vi "setMagnet.vi"(4 "Mode":T2, 6 "Axis":T1=enum."Z", 8 "error in (no error)":errorcluster, 9 "Target Rate (T/min)":dbl, 10 "Target Field (T)":dbl, 11 "Instrument.Cryostat in":refnum<class "Instrument.Cryostat.lvclass">) -> (0 "error out":errorcluster, 3 "Instrument.Cryostat out":refnum<class "Instrument.Cryostat.lvclass">)   [LabVIEW 2019, in "Instrument.Cryostat.lvclass"]
uses:
  Instrument.Cryostat.lvclass
  Typedefs/Magnet Mode--Enum.ctl
  Typedefs/Magnet Axis--Enum.ctl
  Typedefs/setMagnet--cluster.ctl
  Typedefs/Cryostat.commands--enum.ctl
  00381b7c-8845-4057-acc0-7767fffcdb05.vi
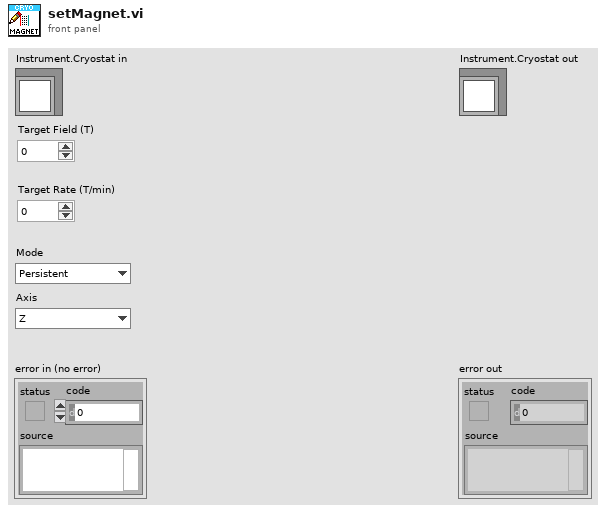
[diagram p1: front panel]
types:
  T1 = typedef "Instrument.Cryostat.lvclass/Magnet Axis--Enum.ctl" = enum16{"X", "Y", "Z"}
  T2 = typedef "Instrument.Cryostat.lvclass/Magnet Mode--Enum.ctl" = enum16{"Persistent", "Driven"}
  T3 = typedef "Instrument.Cryostat.lvclass/Cryostat.commands--enum.ctl" = enum16{"getLN2Level", "getLHeLevel", "getMagnet", "getMagnetVector", "setMagnet", "setMagnetVector", "getAngle", "setAngle", "getTemperature", "setTemperature", "getHeater", "setHeater", "getChamber", "setChamber", ""}
  T4 = typedef "Instrument.Cryostat.lvclass/setMagnet--cluster.ctl" = cluster{"field":dbl, "rate":dbl, "axis":T1, "mode":T2}
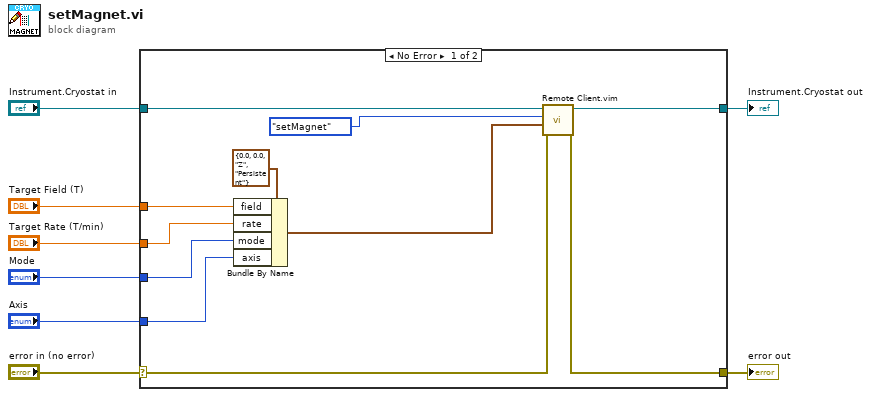
[diagram p0: block diagram]
diagram:
  n1 = case shown="No Error" "error in (no error)" {
    selector: "error in (no error)" -> [w9 w21]
    tunnel: [w15 w21] -> w7
    tunnel: [w12 w20] -> w5
    tunnel: "Instrument.Cryostat in" -> [w10 w20]
    tunnel: "Target Field (T)" -> [w18 _]
    tunnel: "Target Rate (T/min)" -> [w17 _]
    tunnel: "Axis" -> [w13 _]
    tunnel: "Mode" -> [w16 _]
    frame No Error {
      n2 = Bundle By Name(cluster=T4 {"field"=0.0, "rate"=0.0, "axis"=enum."Z", "mode"=enum."Persistent"} ("Set Magnet Field"), "field"=w18, "rate"=w17, "mode"=w16, "axis"=w13) -> (w14:T4)
      n3 = call "Remote Client.vim"("error in (no error)"=w9, "Data in"=w14, "Command in"=Cryostat.commands--enum."setMagnet" ("commands"), "Instrument in"=w10) -> ("error out"=w15:errorcluster, "Instrument out"=w12:refnum<class "Instrument.Cryostat.lvclass">)  [unwired: 4 in, 2 out]
    }
    frame Error {
    }
  }
  "error out" <- w7
  "Instrument.Cryostat out" <- w5
